vi "set_tip_tilt_piezos.vi"() -> ()   [LabVIEW 2016]
panel:
  in  "Number of steps":i32
  in  "Stop Volt (V)":dbl
  in  "Start Volt (V)":dbl
  in  "direction (x,y,z)":string
  in  "Max Volt (V)":dbl
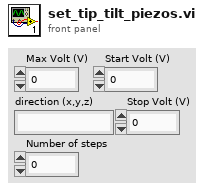
[diagram p1: front panel]
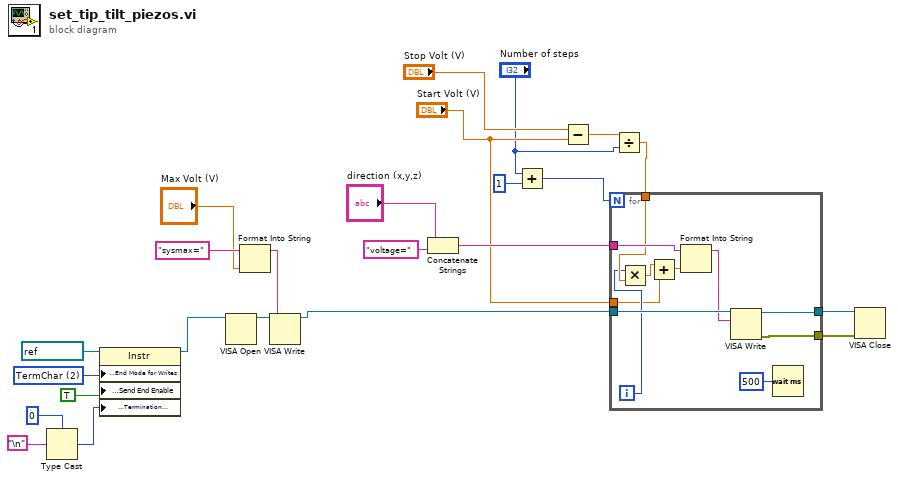
[diagram p0: block diagram]
diagram:
  w21 = u16 2 items=["None", "Last Bit", "TermChar", "Break"] ("Serial Settings:End Mode for Writes")
  n1 = Type Cast(type=u8 0, x="\n") -> (*(type *) &x=w16:u8)
  n2 = property class="Instr"(reference=refnum<visa-resource-name> "COM6" ("VISA resource name"), "Serial Settings:End Mode for Writes"=w21, "Message Based Settings:Send End Enable"=TRUE, "Message Based Settings:Termination Character"=w16) -> (reference out=w19:refnum<visa-resource-name>)  [unwired: 1 in, 1 out]
  n3 = VISA Open(VISA resource name=w19) -> (VISA resource name=w15:refnum<visa-resource-name>)  [unwired: 4 in, 1 out]
  n4 = Format Into String(initial string="sysmax=" ("write buffer"), "Max Volt (V)") -> (resulting string=w12:string)  [unwired: 2 in, 1 out]
  n5 = VISA Write(VISA resource name=w15, write buffer=w12) -> (VISA resource name out=w11:refnum<visa-resource-name>)  [unwired: 1 in, 2 out]
  n6 = Concatenate Strings("direction (x,y,z)", "voltage=" ("string")) -> (w8:string)
  n7 = Add(x="Number of steps", y=1) -> (x+y=w2:i32)
  n8 = Subtract(x="Stop Volt (V)", y="Start Volt (V)") -> (x-y=w6:dbl)
  n9 = Divide(x=w6, y="Number of steps") -> (x/y=w5:dbl)
  n10 = for {
    N: w2 -> [_]
    tunnel: [w34] -> w23
    tunnel: w8 -> [w32]
    tunnel: w11 -> [w33]
    tunnel: [w35] -> w24
    tunnel: w5 -> [w28]
    tunnel: "Start Volt (V)" -> [w26]
    i -> [w27]
    n11 = Multiply(x=w27, y=w28) -> (x*y=w29:dbl)
    n12 = Add(x=w29, y=w26) -> (x+y=w30:dbl)
    n13 = Format Into String(initial string=w32, w30) -> (resulting string=w31:string)  [unwired: 2 in, 1 out]
    n14 = VISA Write(VISA resource name=w33, write buffer=w31) -> (VISA resource name out=w35:refnum<visa-resource-name>, error out=w34:errorcluster)  [unwired: 1 in, 1 out]
    n15 = Wait (ms)(milliseconds to wait=u32 500) -> ()  [unwired: 1 out]
  }
  n16 = VISA Close(VISA resource name=w24, error in (no error)=w23) -> ()  [unwired: 1 out]
